vi "Init_SSH.vi"(10 "Raspberry Pi":T1={"IP Address"="raspberrypi.local", "Username"="pi", "password"="raspberry"}, 11 "Python version":string="3.7") -> (0 "error out":errorcluster, 1 "Console out":string, 3 "Python":T2)   [LabVIEW 2020]
uses:
  PythonCtrl.ctl
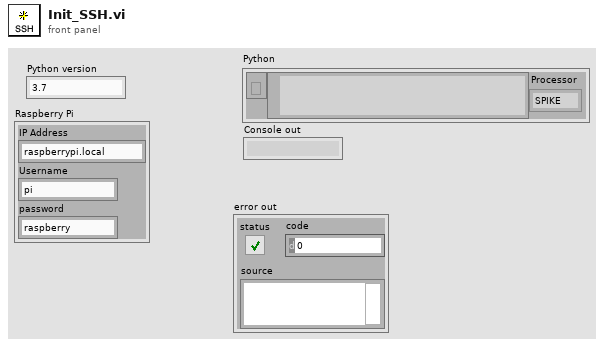
[diagram p1: front panel]
types:
  T1 = cluster{"IP Address":string, "Username":string, "password":string}
  T2 = typedef "PythonCtrl.ctl" = cluster{"session":refnum<k35>, "PyPath":path, "Processor":enum16{"SPIKE", "Pi"}}
  T3 = cluster{"session out":refnum<k35>, "appended path":path, i32}
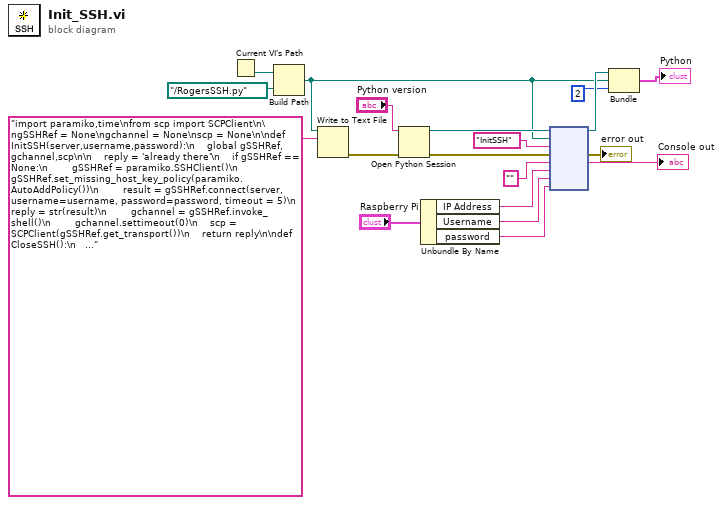
[diagram p0: block diagram]
diagram:
  n1 = Current VI's Path() -> (path=w3:path)
  n2 = Build Path(base path=w3, name or relative path=path "../RogersSSH.py" ("base path")) -> (appended path=w9:path)
  n3 = Write to Text File(file (use dialog)=w9, text="import paramiko,time\nfrom scp import SCPClient\n\ngSSHRef = None\ngchannel = None\nscp = None\n\ndef InitSSH(server,username,password):\n    global gSSHRef, gchannel,scp\n\n    reply = 'already there'\n    if gSSHRef == None:\n        gSSHRef = paramiko.SSHClient()\n        gSSHRef.set_missing_host_key_policy(paramiko.AutoAddPolicy())\n        result = gSSHRef.connect(server, username=username, password=password, timeout = 5)\n        reply = str(result)\n        gchannel = gSSHRef.invoke_shell()\n        gchannel.settimeout(0)\n    scp = SCPClient(gSSHRef.get_transport())\n    return reply\n\ndef CloseSSH():\n    if gchannel != None:\n        gchannel.close()\n    if gSSHRef != None:\n        gSSHRef.close()\n    if scp != None:\n        scp.close()\n    return('done')\n\ndef WriteSSH(string):\n    global gSSHRef, gchannel,scp\n    reply = 'no reference'\n    if gSSHRef != None:\n        reply = 'no file'\n        if gchannel != None:\n            size = gchannel.send(string.encode())\n            reply = str(size)\n    return reply\n\ndef ReadSSH():\n    global gSSHRef, gchannel,scp\n    reply = 'no reference'\n    if gSSHRef != None:\n        reply = 'no file'\n        if gchannel != None:\n            reply = ''\n            if gchannel.recv_ready():\n                reply = gchannel.recv(9999).decode()\n\n    return(reply)\n\ndef WriteWaitReadSSH(string,char,timeout=10000):\n     global gSSHRef, gchannel,scp\n     reply = ReadSSH()\n     WriteSSH(string)\n     n = int(timeout/10)\n     for i in range(n):\n         ans = ReadSSH()\n         reply = reply + ans\n         if ans.find(char) >= 0:\n             #print(ans)\n             return reply\n         time.sleep(0.01)\n     return reply\n\ndef scp_get(name):\n     try:\n          scp.get(name)\n          return 'get succeeded\\n'\n     except Exception as e:\n          return  'scp.get('+name+')\\n' +str(e)\n\ndef scp_put(source, dest):\n     try:\n          scp.put(source, dest)\n          return 'scp.put('+source+','+dest+')\\n' +'put succeeded\\n'\n     except Exception as e:\n          return str(e)\n\ndef scp_put_all(source, dest):\n     try:\n          scp.put(source, recursive = True, remote_path = dest)\n          return 'put succeeded\\n'\n     except Exception as e:\n          return str(e)\n" ("name or relative path")) -> (error out=w19:errorcluster)  [unwired: 2 in, 2 out]
  n4 = Open Python Session(python version="Python version", 3:w19) -> (session out=w10:refnum<k35>, error out=w6:errorcluster)  [unwired: 1 in]
  n5 = Unbundle By Name("Raspberry Pi") -> ("IP Address"=w13:string, "Username"=w12:string, "password"=w11:string)
  n6 = node(w10, w9, "InitSSH" ("function name"), w6, "" ("function name"), w13, w12, w11) -> (w16:refnum<k35>, →"error out":errorcluster, →"Console out":string)  [unwired: 3 in, 2 out]
  n7 = Bundle("session out"=w16, "appended path"=w9, 2) -> (→"Python":T3)  [unwired: 1 in]
